vi "Get Devicetype Variables.vi"(8 "error in":errorcluster, 11 "string":string) -> (0 "error out":errorcluster, 2 "Sorted List":string[](array[string]), 3 "substring":string)   [LabVIEW 2013]
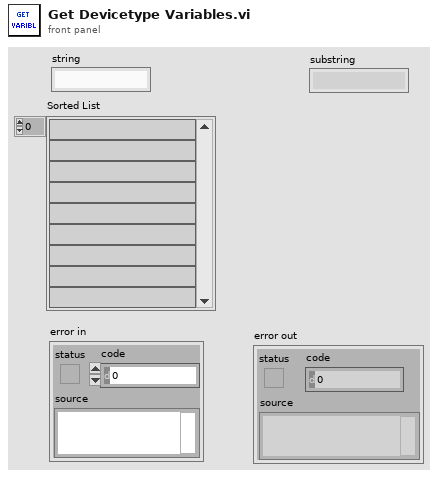
[diagram p1: front panel]
types:
  T1 = typedef "mysql_authentication.ctl" = cluster{"User":string, "Password":string, "Database":string}
  T2 = cluster{"Port":u16, "IP Address":string, "Authentication":T1}
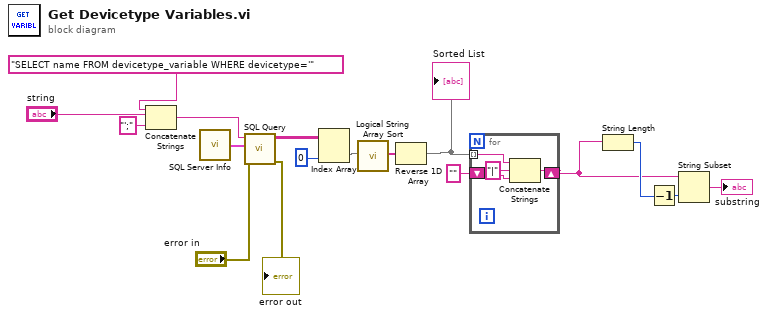
[diagram p0: block diagram]
diagram:
  n1 = Concatenate Strings("SELECT name FROM devicetype_variable WHERE devicetype='", "string", "';" ("string")) -> (w4:string)
  n2 = call "SQL Server Info.vi"() -> ("SQL Server Info"=w13:T2)
  n3 = call "SQL Query.vi"("error in (no error)"="error in", "SQL Server Info"=w13, "Query"=w4) -> ("error out"=→"error out":errorcluster, "data"=w9:string[][])  [unwired: 7 in]
  n4 = Index Array(array=w9, index (col)=0 ("disabled index (col)")) -> (element=w8:string[])  [unwired: 1 in]
  n5 = call "Logical String Array Sort.vi"("Unsorted List"=w8) -> ("Sorted List"=w1:string[])  [unwired: 18 in]
  n6 = Reverse 1D Array(array=w1) -> (reversed array=w7:string[])
  "Sorted List" <- w7
  n7 = for {
    tunnel: w7 -> [w21] mode=indexing
    shift-right: [w19] -> w16
    shift-left: "" -> [w18]
    n8 = Concatenate Strings(w21, "|" ("string"), w18) -> (w19:string)
  }
  n9 = String Length(string=w16) -> (length=w17:i32)
  n10 = Decrement(x=w17) -> (x-1=w15:i32)
  n11 = String Subset(string=w16, length (rest)=w15) -> (substring=→"substring":string)  [unwired: 1 in]
